vi "Guia-1.vi"() -> ()   [LabVIEW 2014]
doc: "Newport Motion Controler\nThis VI test a Group\n\nAndré Romero - 2022\nandretec@ifsc.usp.br"
uses:
  <vilib>/Platform/TimedLoop/XDataNode/timing_clust.ctl
  <vilib>/Platform/TimedLoop/XDataNode/nitl_modes.ctl
  <vilib>/Platform/TimedLoop/XDataNode/wakeup.ctl
  <vilib>/Platform/TimedLoop/XDataNode/XDataNode.xnode
  <userlib>/Newport ESP301/Newport ESP301.lvlib
  <vilib>/Platform/TimedLoop/XDataNode/XDNodeRunTimeDep.lvlib
panel:
  in  "Stop Button":bool
  out "error out":errorcluster
  out "Y":dbl format="%.2g"
  out "X":dbl=1.0 format="%.2f"
  out "XY Graph":cluster{dbl[], dbl[]}(graph)
  in  "Velocity":dbl=0.05
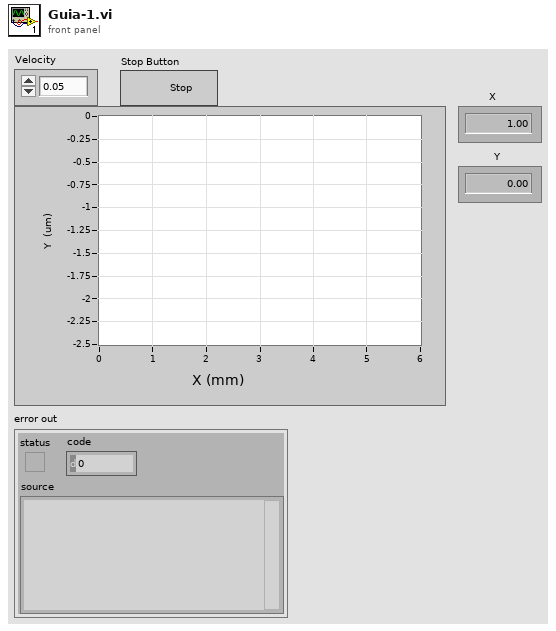
[diagram p1: front panel]
types:
  T1 = typedef "XDNodeRunTimeDep.lvlib/timing_clust.ctl" = cluster{"Expected End [f-1]":u64, "Actual End [f-1]":u64, "Finished Late? [f-1]":bool, "Expected End [i-1]":u64, "Actual End [i-1]":u64, "Finished Late? [i-1]":bool, "Expected Start [i]":u64, "Actual Start [i]":u64, "Expected Start [f]":u64, "Actual Start [f]":u64, "Source Name":string, "Structure Name":string, "Period":i64, "Deadline":i64, "Offset":i64, "Start":i64, "Priority":i32, "Timeout":i32, "Mode":T2, "Wakeup Reason":T3, "Error":errorcluster, "Source Type":string, "Secondary Source Type":string, "Global End Time":u64, "Global Start Time":u64, "Frame Duration":u64, "Iteration Duration":u64, "Assigned CPU":i32, "I/O Scan Engine Mode":u32}
  T2 = typedef "XDNodeRunTimeDep.lvlib/nitl_modes.ctl" = enum32{"No Change", "Process missed periods, maintain original phase", "Discard missed periods, maintain original phase", "Process missed periods, ignore original phase", "Discard missed periods, ignore original phase"}
  T3 = typedef "XDNodeRunTimeDep.lvlib/wakeup.ctl" = enum32{"Normal", "Aborted", "Asynchronous wakeup", "Timing source error", "Timed loop error", "Timeout"}
  T4 = cluster{"first coordonate of arc":dbl, "Second coordonate of arc center":dbl, "arc sweep angle":dbl}
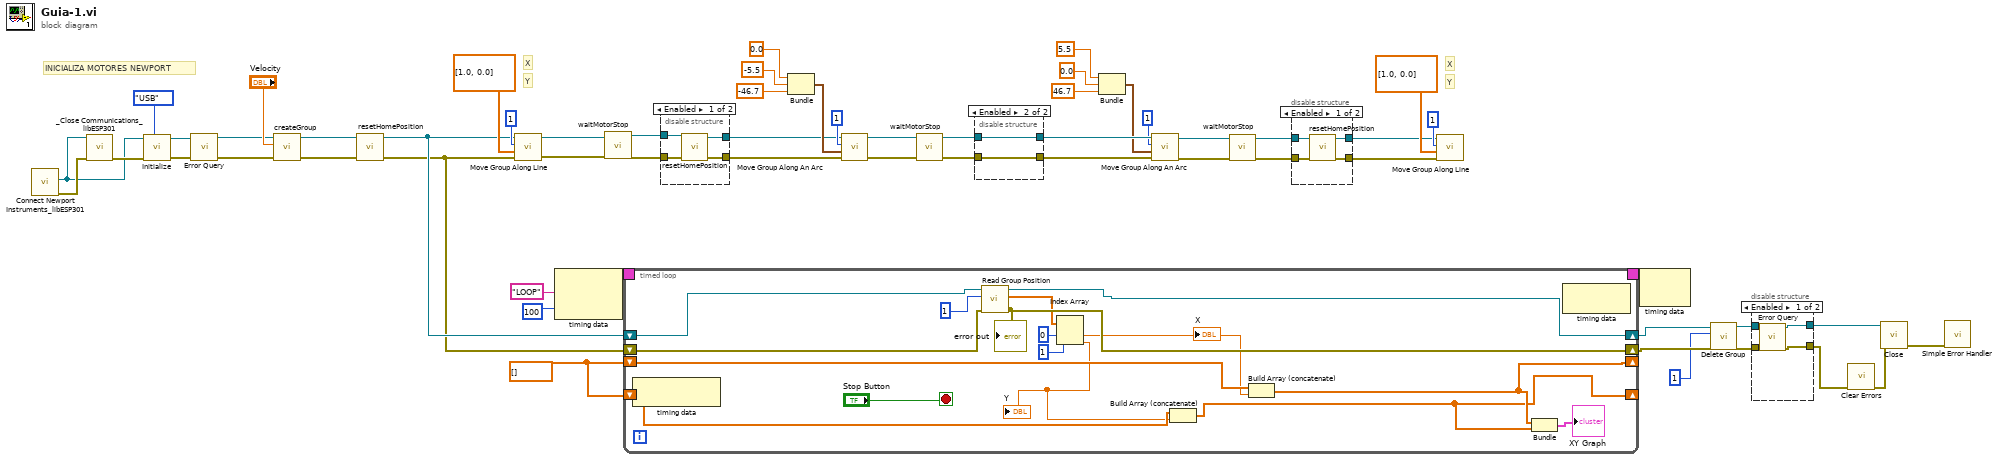
[diagram p0: block diagram]
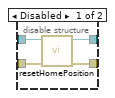
[diagram p4: hidden frame]
diagram:
  w44 = dbl[] []
  # "Y"
  # "X"
  # "Y"
  # "X"
  # "INICIALIZA MOTORES NEWPORT"
  n1 = call <userlib>:"Connect Newport Instruments_libESP301.vi"() -> ("error (duplicate)"=w57:errorcluster, "VISA resource name (duplicate)"=w56:refnum<visa-resource-name>)  [unwired: 7 in, 3 out]
  n2 = call <userlib>:"_Close Communications_libESP301.vi"("Instrument Channel"=w56, "error in (no error)"=w57) -> ("error out"=w59:errorcluster)  [unwired: 13 in]
  n3 = call <userlib>:"Initialize.vi"("VISA resource name"=w56, "error in (no error)"=w59, "Serial Link (RS232)"=enum16{"RS232", "USB"}."USB") -> ("VISA resource name out"=w55:refnum<visa-resource-name>, "error out"=w54:errorcluster)  [unwired: 6 in]
  n4 = call <userlib>:"Error Query.vi"("error in (no error)"=w54, "VISA resource name"=w55) -> ("error out"=w32:errorcluster, "VISA resource name out"=w33:refnum<visa-resource-name>)  [unwired: 2 in, 2 out]
  n5 = call "createGroup.vi"("error in (no error)"=w32, "Velocity"="Velocity", "VISA Refnum in"=w33) -> ("error out"=w4:errorcluster, "VISA Refnum out"=w3:refnum<visa-resource-name>)  [unwired: 7 in]
  n6 = call "resetHomePosition.vi"("error in (no error)"=w4, "VISA Refnum in"=w3) -> ("error out"=w1:errorcluster, "VISA Refnum out"=w2:refnum<visa-resource-name>)  [unwired: 8 in]
  n7 = call <userlib>:"Move Group Along Line.vi"("error in (no error)"=w1, "Position (0 units)"=dbl[] [1.0, 0.0], "Group Number (1)"=1, "VISA resource name"=w2) -> ("error out"=w20:errorcluster, "VISA resource name out"=w21:refnum<visa-resource-name>)  [unwired: 2 in]
  n8 = node-c288("LOOP" ("Structure Name"), i64 100 ("Period")) -> (w48:T1)
  n9 = call "waitMotorStop.vi"("error in (no error)"=w20, "VISA Refnum in"=w21) -> ("error out"=w18:errorcluster, "VISA Refnum out"=w19:refnum<visa-resource-name>)  [unwired: 8 in]
  n10 = timed-loop {
    timing: w48 -> [_]
    timing-out: [_] -> w47
    shift-right: [w70] -> w39
    shift-left: w2 -> [w72]
    shift-right: [w69] -> w38
    shift-left: w1 -> [w71]
    shift-right: [w61] -> _
    shift-left: w44 -> [w75]
    shift-right: [w60] -> _
    shift-left: w44 -> [w74]
    stop <- "Stop Button" stop-if-true
    n11 = node-c288() -> ()  [unwired: 1 in, 1 out]
    n12 = call <userlib>:"Read Group Position.vi"("error in (no error)"=w71, "Group Number (1)"=1, "VISA resource name"=w72) -> ("error out"=w69:errorcluster, "Position (units)"=w66:dbl[], "VISA resource name out"=w70:refnum<visa-resource-name>)  [unwired: 2 in]
    "error out" <- w69
    n13 = Index Array(array=w66, index #1=0 ("index"), index #2=1 ("index")) -> (element #1=w65:dbl, element #2=w64:dbl)
    "Y" <- w64
    "X" <- w65
    n14 = Build Array (concatenate)(w74, w64) -> (w60:dbl[])
    n15 = Build Array (concatenate)(w75, w65) -> (w61:dbl[])
    n16 = Bundle(w61, w60) -> (→"XY Graph":cluster{dbl[], dbl[]})  [unwired: 1 in]
    n17 = node-c288() -> ()  [unwired: 1 in, 1 out]
  }
  n18 = disable-structure shown="Enabled" {
    disable-tunnel: [w81 w83] -> w31
    disable-tunnel: [w80 w82] -> w30
    disable-tunnel: w19 -> [w79 w83]
    disable-tunnel: w18 -> [w78 w82]
    frame Enabled {
      n19 = call "resetHomePosition.vi"("error in (no error)"=w78, "VISA Refnum in"=w79) -> ("error out"=w80:errorcluster, "VISA Refnum out"=w81:refnum<visa-resource-name>)  [unwired: 8 in]
    }
    frame Disabled {
    }
  }
  n20 = Bundle("first coordonate of arc"=0.0, "Second coordonate of arc center"=-5.5, "arc sweep angle"=-46.7) -> (w49:T4)  [unwired: 1 in]
  n21 = call <userlib>:"Move Group Along An Arc.vi"("error in (no error)"=w30, "Arc  Parameters"=w49, "Group Number (1)"=1, "VISA resource name"=w31) -> ("error out"=w26:errorcluster, "VISA resource name out"=w27:refnum<visa-resource-name>)  [unwired: 2 in]
  n22 = call "waitMotorStop.vi"("error in (no error)"=w26, "VISA Refnum in"=w27) -> ("error out"=w25:errorcluster, "VISA Refnum out"=w24:refnum<visa-resource-name>)  [unwired: 8 in]
  n23 = disable-structure shown="Enabled" {
    disable-tunnel: [w87 w89] -> w29
    disable-tunnel: [w86 w88] -> w28
    disable-tunnel: w25 -> [w85 w88]
    disable-tunnel: w24 -> [w84 w89]
    frame Disabled {
      n24 = call "resetHomePosition.vi"("error in (no error)"=w85, "VISA Refnum in"=w84) -> ("error out"=w86:errorcluster, "VISA Refnum out"=w87:refnum<visa-resource-name>)  [unwired: 8 in]
    }
    frame Enabled {
    }
  }
  n25 = Bundle("first coordonate of arc"=5.5, "Second coordonate of arc center"=0.0, "arc sweep angle"=46.7) -> (w13:T4)  [unwired: 1 in]
  n26 = call <userlib>:"Move Group Along An Arc.vi"("error in (no error)"=w28, "Arc  Parameters"=w13, "Group Number (1)"=1, "VISA resource name"=w29) -> ("error out"=w8:errorcluster, "VISA resource name out"=w7:refnum<visa-resource-name>)  [unwired: 2 in]
  n27 = call "waitMotorStop.vi"("error in (no error)"=w8, "VISA Refnum in"=w7) -> ("error out"=w5:errorcluster, "VISA Refnum out"=w6:refnum<visa-resource-name>)  [unwired: 8 in]
  n28 = disable-structure shown="Enabled" {
    disable-tunnel: [w93 w95] -> w10
    disable-tunnel: [w92 w94] -> w9
    disable-tunnel: w6 -> [w91 w95]
    disable-tunnel: w5 -> [w90 w94]
    frame Enabled {
      n29 = call "resetHomePosition.vi"("error in (no error)"=w90, "VISA Refnum in"=w91) -> ("error out"=w92:errorcluster, "VISA Refnum out"=w93:refnum<visa-resource-name>)  [unwired: 8 in]
    }
    frame Disabled {
    }
  }
  n30 = call <userlib>:"Move Group Along Line.vi"("error in (no error)"=w9, "Position (0 units)"=dbl[] [1.0, 0.0], "Group Number (1)"=1, "VISA resource name"=w10) -> ()  [unwired: 2 in, 2 out]
  n31 = node-c288(w47) -> ()  [unwired: 1 out]
  n32 = call <userlib>:"Delete Group.vi"("error in (no error)"=w38, "Group Number (1)"=1, "VISA resource name"=w39) -> ("error out"=w42:errorcluster, "VISA resource name out"=w43:refnum<visa-resource-name>)  [unwired: 3 in]
  n33 = disable-structure shown="Enabled" {
    disable-tunnel: w43 -> [w99 w101]
    disable-tunnel: w42 -> [w98 w100]
    disable-tunnel: [w97 w101] -> w41
    disable-tunnel: [w96 w100] -> w36
    frame Enabled {
      n34 = call <userlib>:"Error Query.vi"("error in (no error)"=w98, "VISA resource name"=w99) -> ("error out"=w96:errorcluster, "VISA resource name out"=w97:refnum<visa-resource-name>)  [unwired: 2 in, 2 out]
    }
    frame Disabled {
    }
  }
  n35 = call <vilib>:"Clear Errors.vi"("error in (no error)"=w36) -> ("error out"=w35:errorcluster)  [unwired: 5 in, 1 out]
  n36 = call <userlib>:"Close.vi"("error in (no error)"=w35, "VISA resource name"=w41) -> ("error out"=w40:errorcluster)  [unwired: 9 in]
  n37 = call <vilib>:"Simple Error Handler.vi"("error in (no error)"=w40) -> ()  [unwired: 4 in, 5 out]
